vi "View.vi"(8 "error in (no error)":errorcluster) -> (0 "error out":errorcluster)   [LabVIEW 2019, in "STS_LTRV.lvlib"]
uses:
  STS_LTRV.lvlib
  Queue Driver/Queue Operation.ctl
  TypeDefs/Event Handler/Operation.ctl
  TypeDefs/UI Data.ctl
  TypeDefs/Publish Data.ctl
  TypeDefs/NumericLimit Data.ctl
  <vilib>/Utility/miscctls.llb/LVRowAndColumnTypeDef.ctl
  Queue Driver/Queue Driver.lvlib
panel:
  in  "Group Results by UUT":bool=TRUE
  in  "Max UUTs to Store":i32
  out "Diaplay Table":string[][](table)
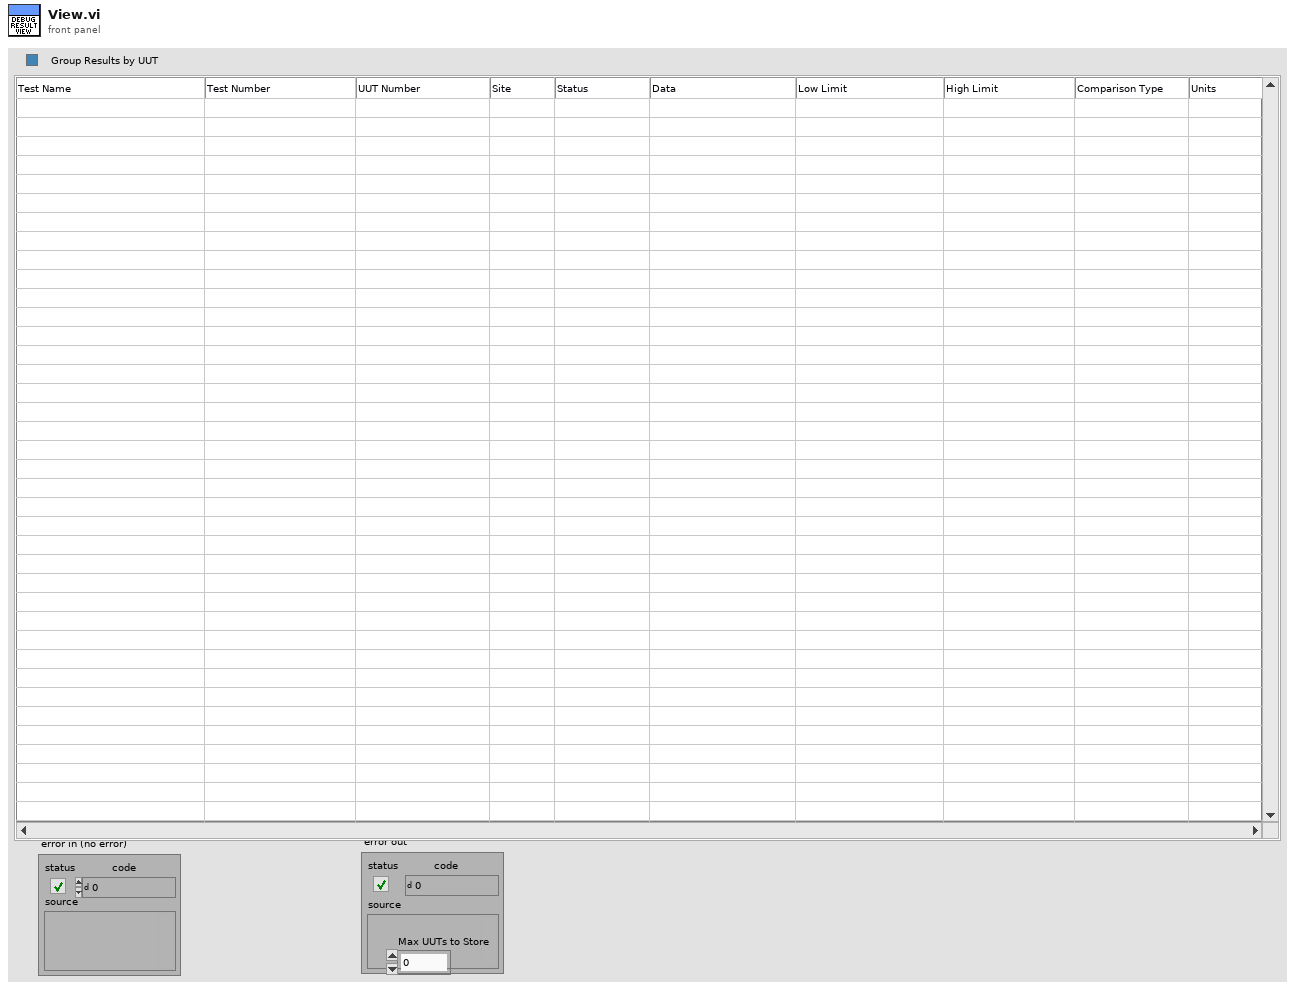
[diagram p1: front panel]
types:
  T1 = typedef "STS_LTRV.lvlib/UI Data.ctl" = cluster{"Order":u64, "Publish Data":T2}
  T2 = typedef "STS_LTRV.lvlib/Publish Data.ctl" = cluster{"TestName":string, "TestNumber":dbl, "Status":string, "UUT.SerialNumber":string, "Site":dbl, "NumericLimit":T3}
  T3 = typedef "STS_LTRV.lvlib/NumericLimit Data.ctl" = cluster{"Data":dbl, "LowLimit":dbl, "HighLimit":dbl, "ComparisonType":string, "Units":string}
  T4 = typedef "STS_LTRV.lvlib/Operation.ctl" = enum16{"Initilize", "Get Reference", "Publish", "Destroy"}
  T5 = cluster{"Data":variant, "Next Order Id":u64, "Max UUTs to Store":i32, "Group Results by UUT":bool}
  T6 = typedef "Queue Driver.lvlib/Queue Operation.ctl" = enum16{"Create", "Enqueue", "EnqueueN", "Dequeue", "Flush", "Destroy"}
  T7 = typedef "LVRowAndColumnTypeDef.ctl" = cluster{"Row":i32, "Column":i32}
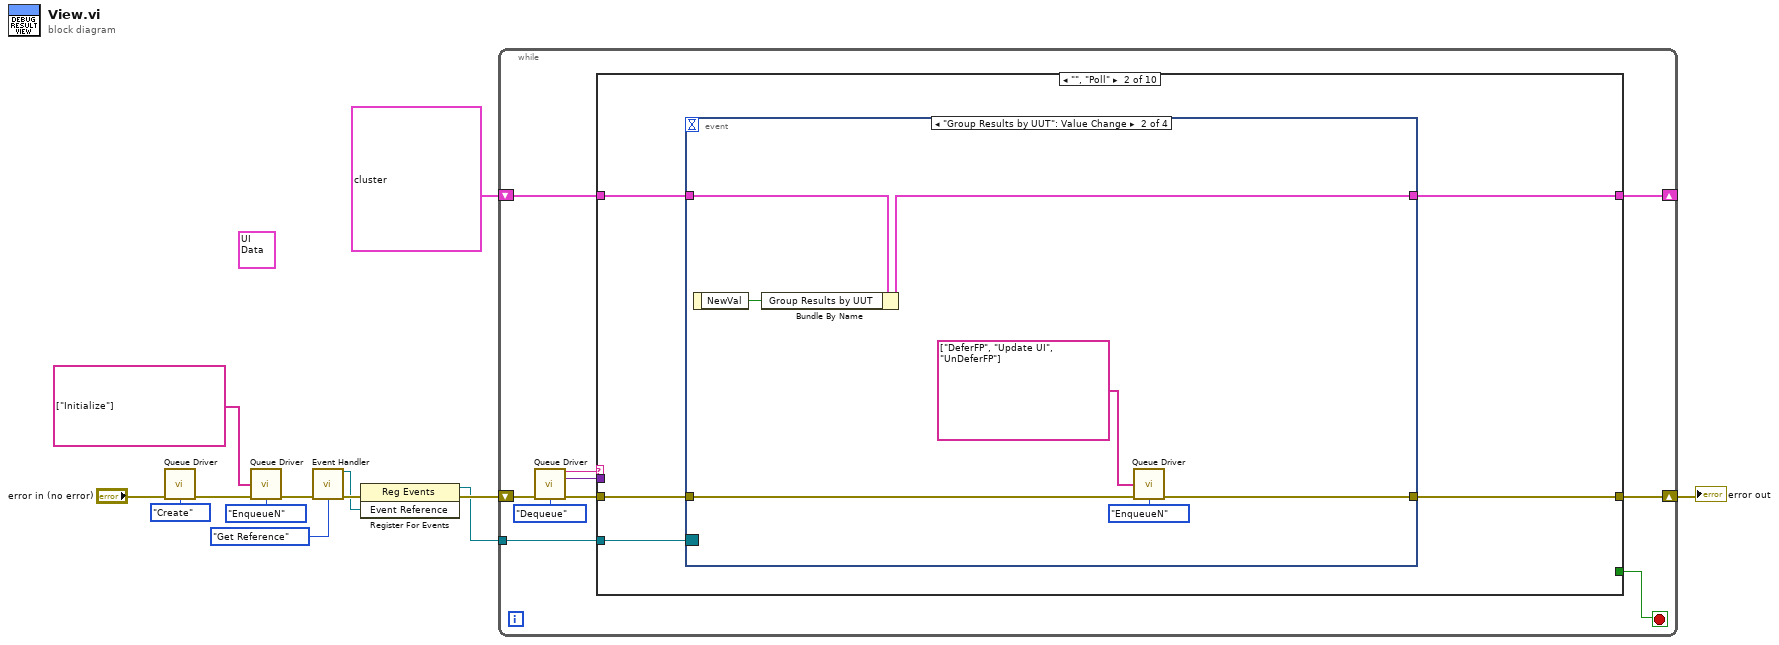
[diagram p0: block diagram]
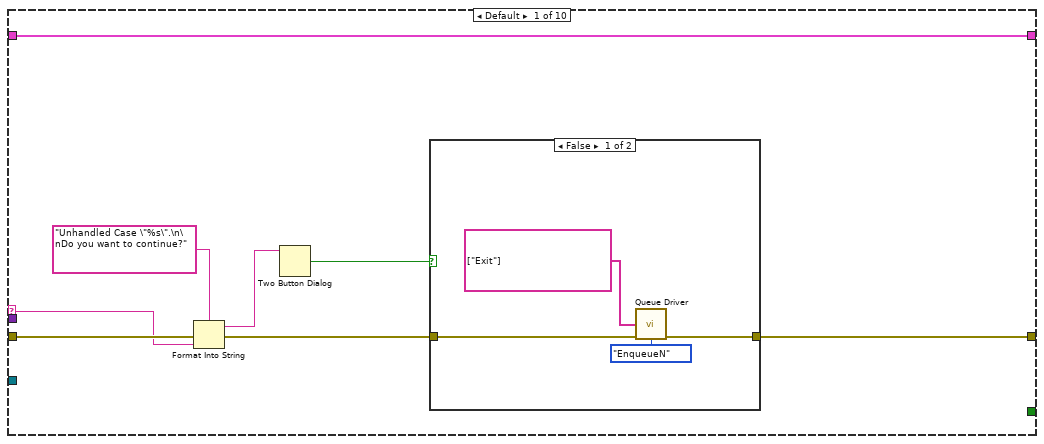
[diagram p2: hidden frame]
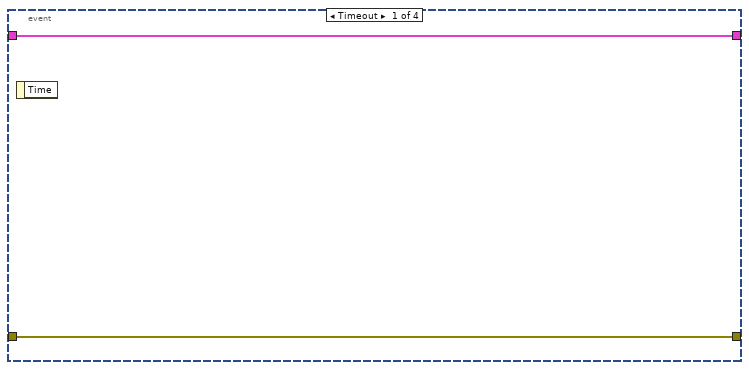
[diagram p4: hidden frame]
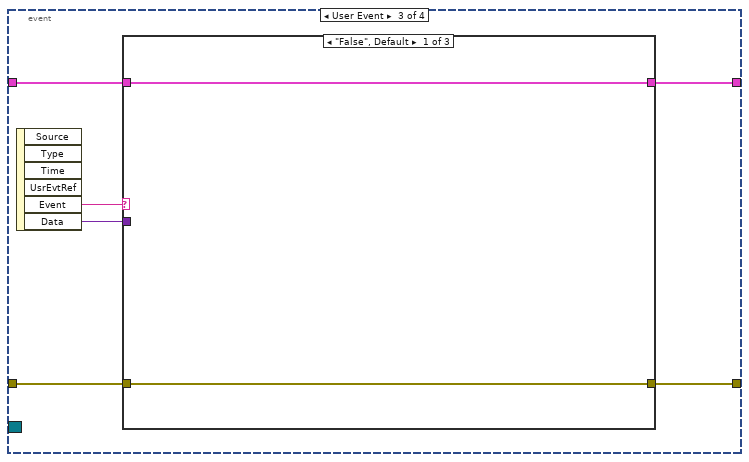
[diagram p5: hidden frame]
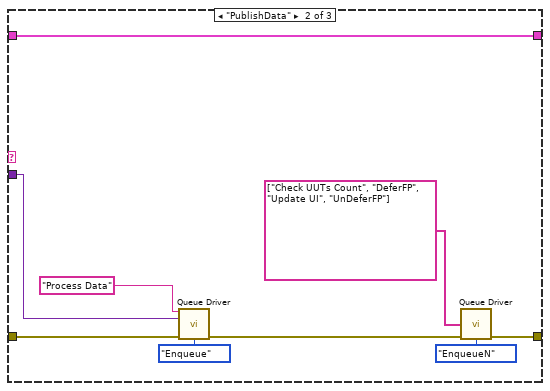
[diagram p6: hidden frame]
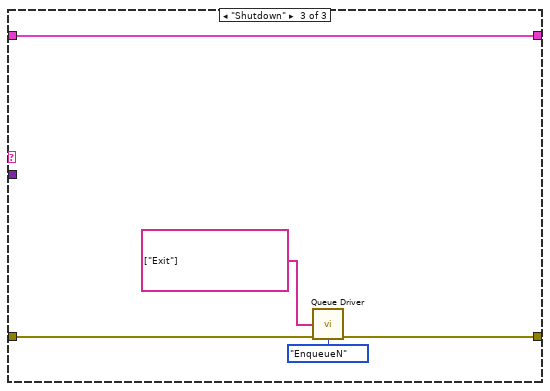
[diagram p7: hidden frame]
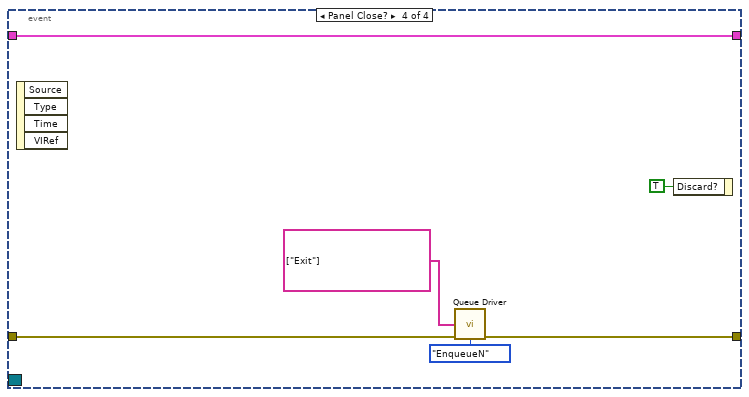
[diagram p8: hidden frame]
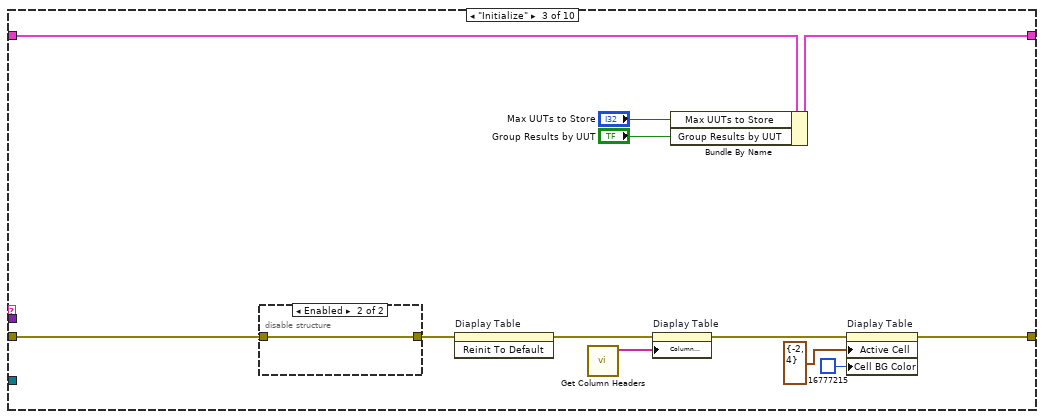
[diagram p9: hidden frame]
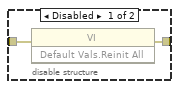
[diagram p10: hidden frame]
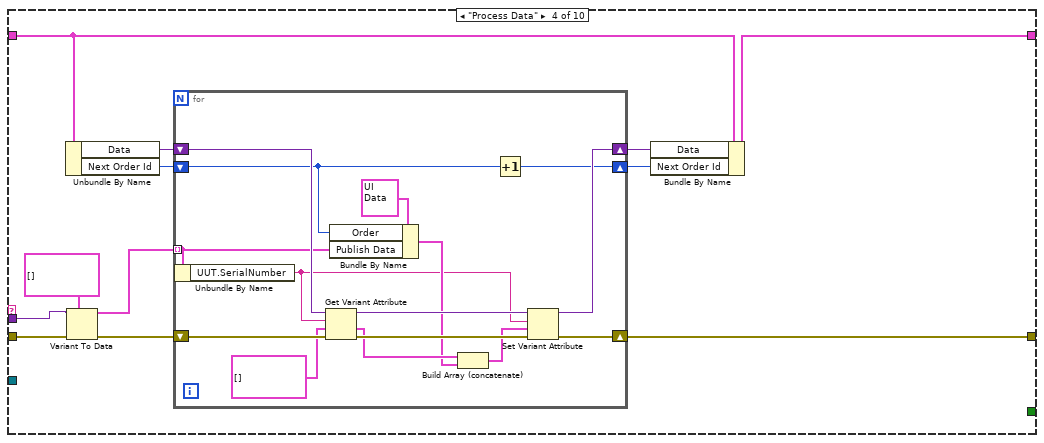
[diagram p11: hidden frame]
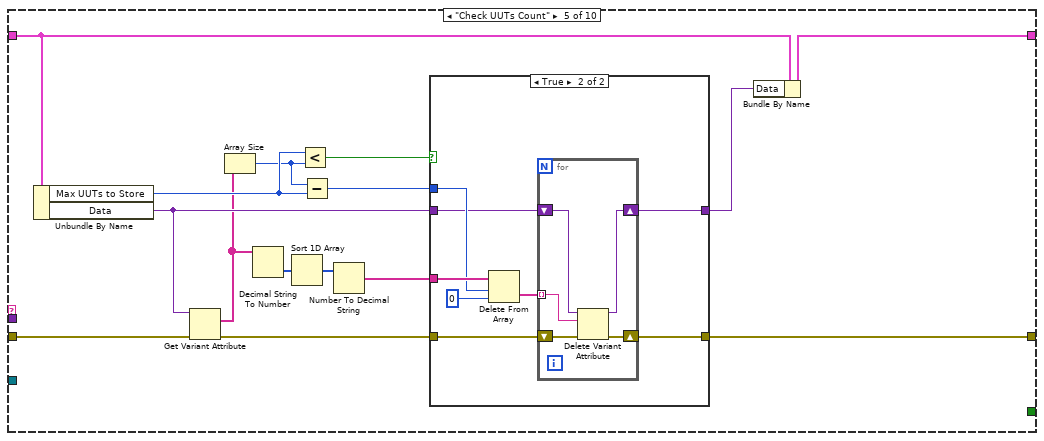
[diagram p12: hidden frame]
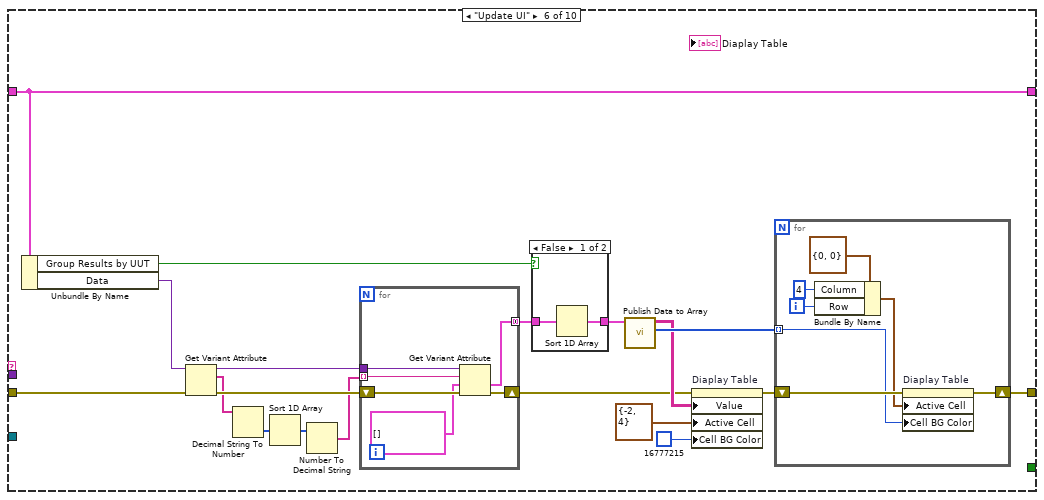
[diagram p14: hidden frame]
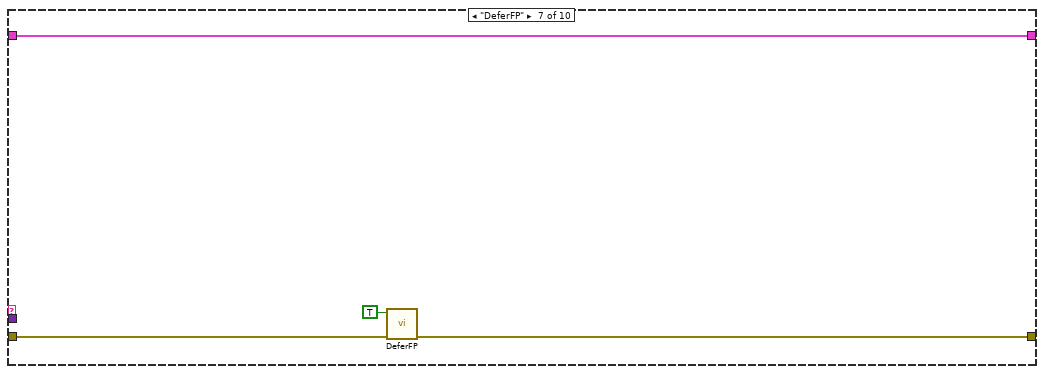
[diagram p16: hidden frame]
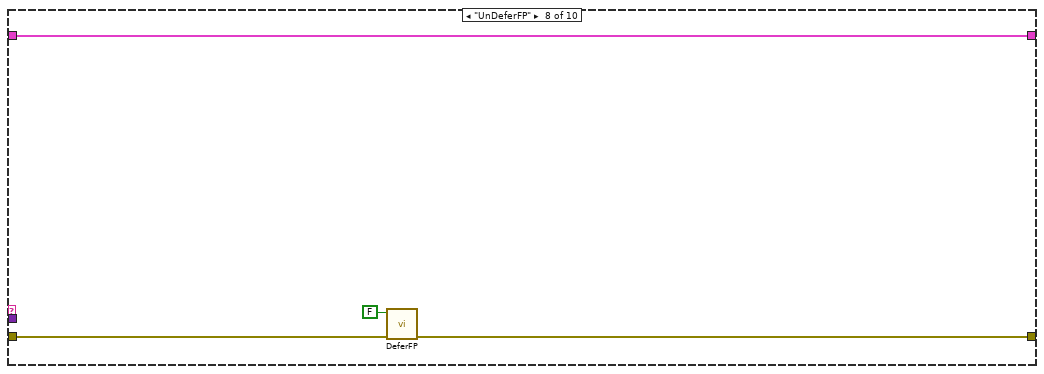
[diagram p17: hidden frame]
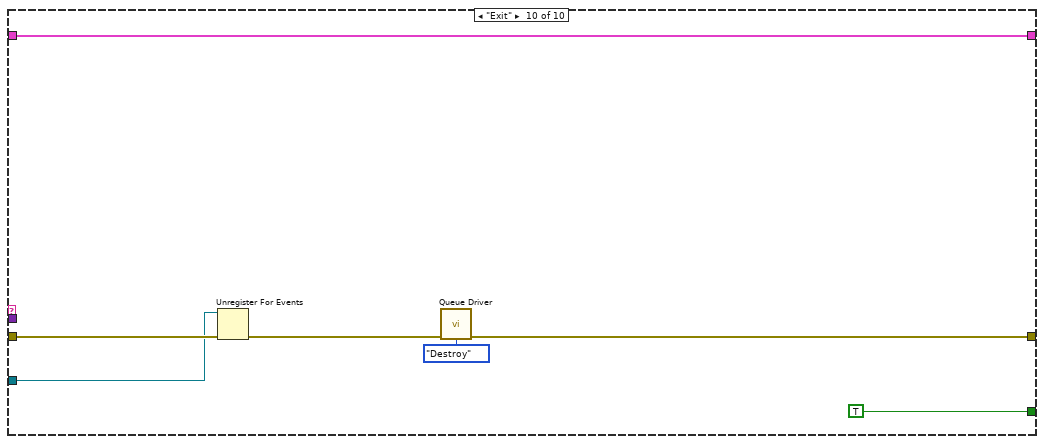
[diagram p19: hidden frame]
diagram:
  (unwired) T1 {"Order"=0, "Publish Data"={"TestName"="", "TestNumber"=0.0, "Status"="", "UUT.SerialNumber"="", "Site"=0.0, "NumericLimit"={"Data"=0.0, "LowLimit"=0.0, "HighLimit"=0.0, "ComparisonType"="", "Units"=""}}}
  n1 = call "Queue Driver.vi"("error in (no error)"="error in (no error)", "Queue Operation"=Queue_Operation."Create") -> ("error out"=w10:errorcluster)  [unwired: 11 in, 2 out]
  n2 = call "Queue Driver.vi"("EnqueueN States"=string[] ["Initialize"], "error in (no error)"=w10, "Queue Operation"=Queue_Operation."EnqueueN") -> ("error out"=w6:errorcluster)  [unwired: 10 in, 2 out]
  n3 = call "Event Handler.vi"("error in (no error)"=w6, "Operation"=Operation."Get Reference") -> ("Event Reference"=w2:refnum<user-event>, "error out"=w4:errorcluster)  [unwired: 12 in]
  n4 = register-events(error in=w4, w2) -> (reference out=w1:refnum<event-registration>, error out=w3:errorcluster)  [unwired: 1 in]
  n5 = while {
    shift-right: [w17] -> _
    shift-left: T5 {"Data"=variant, "Next Order Id"=0, "Max UUTs to Store"=0, "Group Results by UUT"=FALSE} -> [w19]
    shift-right: [w18] -> w7
    shift-left: w3 -> [w22]
    tunnel: w1 -> [w15]
    stop <- w16 stop-if-true
    n6 = call "Queue Driver.vi"("error in (no error)"=w22, "Queue Operation"=Queue_Operation."Dequeue") -> ("State Out"=w20:string, "Data Out"=w14:variant, "error out"=w21:errorcluster)  [unwired: 11 in]
    n7 = case shown="\"\", \"Poll\"" w20 {
      selector: w20 -> [w29 _ _ _ _ _ _ _ _ _]
      tunnel: w21 -> [w30 w41 w90 w105 w135 w168 w186 w190 w195 w197]
      tunnel: w19 -> [w31 w40 w86 w94 w127 w169 w189 w193 w194 w202]
      tunnel: [w25 w39 w80 w101 w130 w156 w187 w191 w195 w200] -> w18
      tunnel: [w31 w38 w87 w95 w128 w169 w189 w193 w194 w202] -> w17
      tunnel: [_ _ _ _ _ _ _ _ _ TRUE] -> w16
      tunnel: w15 -> [_ w37 _ _ _ _ _ _ _ w196]
      tunnel: w14 -> [_ _ _ w104 _ _ _ _ _ _]
      frame Default {
        n8 = Format Into String(format string="Unhandled Case \"%s\".\n\nDo you want to continue?", error in=w30, w29) -> (resulting string=w27:string, error out=w26:errorcluster)  [unwired: 1 in]
        n9 = Two Button Dialog(message=w27) -> (T button?=w24:bool)  [unwired: 2 in]
        n10 = case shown="False" w24 {
          tunnel: w26 -> [w34 w36]
          tunnel: [w33 w36] -> w25
          frame False {
            n11 = call "Queue Driver.vi"("EnqueueN States"=string[] ["Exit"], "error in (no error)"=w34, "Queue Operation"=Queue_Operation."EnqueueN") -> ("error out"=w33:errorcluster)  [unwired: 10 in, 2 out]
          }
          frame True {
          }
        }
      }
      frame "", "Poll" {
        n12 = event shown="[1] \"Group Results by UUT\": Value Change" {
          selector: w37 -> [_ _ _ _]
          dyn-events: _ -> [_ _ _ _]
          timeout: _ -> [_ _ _ _]
          tunnel: w41 -> [w43 w44 w55 w73]
          tunnel: w40 -> [w42 w49 w52 w78]
          tunnel: [w43 w45 w56 w74] -> w39
          tunnel: [w42 w50 w51 w78] -> w38
          event Timeout {
            n13 = event-data() -> ()  [unwired: 1 in, 1 out]
          }
          event "Group Results by UUT": Value Change {
            n14 = event-data() -> ("NewVal"=w48:bool)  [unwired: 1 in]
            n15 = Bundle By Name(cluster=w49, "Group Results by UUT"=w48) -> (w50:T5)
            n16 = call "Queue Driver.vi"("EnqueueN States"=string[] ["DeferFP", "Update UI", "UnDeferFP"], "error in (no error)"=w44, "Queue Operation"=Queue_Operation."EnqueueN") -> ("error out"=w45:errorcluster)  [unwired: 10 in, 2 out]
          }
          event User Event {
            n17 = event-data() -> ("Event"=w54:string, "Data"=w53:variant)  [unwired: 1 in, 4 out]
            n18 = case shown="\"False\", Default" w54 {
              tunnel: [w58 w65 w70] -> w56
              tunnel: w55 -> [w58 w62 w69]
              tunnel: w53 -> [_ w60 _]
              tunnel: w52 -> [w57 w64 w68]
              tunnel: [w57 w64 w68] -> w51
              frame "False", Default {
              }
              frame "PublishData" {
                n19 = call "Queue Driver.vi"("State In"="Process Data", "Data In"=w60, "error in (no error)"=w62, "Queue Operation"=Queue_Operation."Enqueue") -> ("error out"=w61:errorcluster)  [unwired: 9 in, 2 out]
                n20 = call "Queue Driver.vi"("EnqueueN States"=string[] ["Check UUTs Count", "DeferFP", "Update UI", "UnDeferFP"], "error in (no error)"=w61, "Queue Operation"=Queue_Operation."EnqueueN") -> ("error out"=w65:errorcluster)  [unwired: 10 in, 2 out]
              }
              frame "Shutdown" {
                n21 = call "Queue Driver.vi"("EnqueueN States"=string[] ["Exit"], "error in (no error)"=w69, "Queue Operation"=Queue_Operation."EnqueueN") -> ("error out"=w70:errorcluster)  [unwired: 10 in, 2 out]
              }
            }
          }
          event Panel Close? {
            n22 = event-data() -> ()  [unwired: 1 in, 4 out]
            n23 = call "Queue Driver.vi"("EnqueueN States"=string[] ["Exit"], "error in (no error)"=w73, "Queue Operation"=Queue_Operation."EnqueueN") -> ("error out"=w74:errorcluster)  [unwired: 10 in, 2 out]
            n24 = event-data("Discard?"=TRUE) -> ()  [unwired: 1 in, 1 out]
          }
        }
      }
      frame "Initialize" {
        n25 = disable-structure shown="Enabled" {
          disable-tunnel: w90 -> [w92 w93]
          disable-tunnel: [w91 w93] -> w89
          frame Disabled {
            n26 = invoke class="VI" method="Default Vals.Reinit All"(error in=w92) -> (error out=w91:errorcluster)  [unwired: 2 in, 2 out]
          }
          frame Enabled {
          }
        }
        n27 = invoke on="Diaplay Table" class="Tbl (strict)" method="Reinit To Default"(error in=w89) -> (error out=w84:errorcluster)  [unwired: 2 in, 2 out]
        n28 = call "Get Column Headers.vi"() -> ("Headers"=w85:string[])  [unwired: 11 in]
        n29 = property on="Diaplay Table" class="Tbl (strict)"(error in=w84, "Column Headers[]"=w85) -> (error out=w81:errorcluster)  [unwired: 1 in, 1 out]
        n30 = Bundle By Name(cluster=w86, "Max UUTs to Store"="Max UUTs to Store", "Group Results by UUT"="Group Results by UUT") -> (w87:T5)
        n31 = property on="Diaplay Table" class="Tbl (strict)"(error in=w81, "Active Cell"=T7 {"Row"=-2, "Column"=4} ("Active Cell:Active Cell"), "Cell BG Color"=u32 16777215) -> (error out=w80:errorcluster)  [unwired: 1 in, 1 out]
      }
      frame "Process Data" {
        n32 = Unbundle By Name(w94) -> ("Data"=w100:variant, "Next Order Id"=w98:u64)
        n33 = Variant To Data(error in=w105, type=T2[] [] ("Unprocessed Data"), Variant=w104) -> (data=w99:T2[], error out=w102:errorcluster)
        n34 = for {
          shift-right: [w116] -> w101
          shift-left: w102 -> [w120]
          tunnel: w99 -> [w112] mode=indexing
          shift-right: [w108] -> w97
          shift-left: w100 -> [w119]
          shift-right: [w107] -> w96
          shift-left: w98 -> [w113]
          n35 = Unbundle By Name(w112) -> ("UUT.SerialNumber"=w106:string)
          n36 = Get Variant Attribute(Variant=w119, name=w106, default value (empty Variant)=T1[] [], error in=w120) -> (duplicate Variant=w115:variant, value=w111:T1[], error out=w117:errorcluster)  [unwired: 1 out]
          n37 = Bundle By Name(cluster=T1 {"Order"=0, "Publish Data"={"TestName"="", "TestNumber"=0.0, "Status"="", "UUT.SerialNumber"="", "Site"=0.0, "NumericLimit"={"Data"=0.0, "LowLimit"=0.0, "HighLimit"=0.0, "ComparisonType"="", "Units"=""}}} ("Cluster"), "Order"=w113, "Publish Data"=w112) -> (w110:T1)
          n38 = Build Array (concatenate)(w111, w110) -> (w109:T1[])
          n39 = Increment(x=w113) -> (x+1=w107:u64)
          n40 = Set Variant Attribute(Variant=w115, name=w106, value=w109, error in=w117) -> (Variant out=w108:variant, error out=w116:errorcluster)  [unwired: 1 out]
        }
        n41 = Bundle By Name(cluster=w94, "Data"=w97, "Next Order Id"=w96) -> (w95:T5)
      }
      frame "Check UUTs Count" {
        n42 = Unbundle By Name(w127) -> ("Max UUTs to Store"=w134:i32, "Data"=w129:variant)
        n43 = Get Variant Attribute(Variant=w129, error in=w135) -> (names=w124:string[], error out=w131:errorcluster)  [unwired: 2 in, 2 out]
        n44 = Array Size(array=w124) -> (size(s)=w133:i32)
        n45 = Decimal String To Number(string=w124) -> (number=w123:i32[])  [unwired: 2 in, 1 out]
        n46 = Sort 1D Array(array=w123) -> (sorted array=w122:i32[])
        n47 = Less?(x=w134, y=w133) -> (x < y?=w125:bool)
        n48 = Subtract(x=w133, y=w134) -> (x-y=w132:i32)
        n49 = Number To Decimal String(number=w122) -> (decimal integer string=w121:string[])  [unwired: 1 in]
        n50 = case shown="True" w125 {
          tunnel: w121 -> [_ w145]
          tunnel: w132 -> [_ w144]
          tunnel: w131 -> [w137 w142]
          tunnel: [w137 w141] -> w130
          tunnel: w129 -> [w136 w140]
          tunnel: [w136 w138] -> w126
          frame False {
          }
          frame True {
            n51 = Delete From Array(array=w145, length=w144, index=0) -> (deleted portion=w139:string[])  [unwired: 1 out]
            n52 = for {
              shift-right: [w149] -> w141
              shift-left: w142 -> [w150]
              shift-right: [w146] -> w138
              shift-left: w140 -> [w148]
              tunnel: w139 -> [w147] mode=indexing
              n53 = Delete Variant Attribute(4:w150, 6:w147, 7:w148) -> (0:w149:errorcluster, 3:w146:variant)  [unwired: 1 out]
            }
          }
        }
        n54 = Bundle By Name(cluster=w127, "Data"=w126) -> (w128:T5)
      }
      frame "Update UI" {
        n55 = Unbundle By Name(w169) -> ("Group Results by UUT"=w155:bool, "Data"=w167:variant)
        n56 = Get Variant Attribute(Variant=w167, error in=w168) -> (duplicate Variant=w165:variant, names=w154:string[], error out=w166:errorcluster)  [unwired: 2 in, 1 out]
        n57 = Decimal String To Number(string=w154) -> (number=w153:i32[])  [unwired: 2 in, 1 out]
        n58 = Sort 1D Array(array=w153) -> (sorted array=w152:i32[])
        n59 = Number To Decimal String(number=w152) -> (decimal integer string=w151:string[])  [unwired: 1 in]
        n60 = for {
          shift-right: [w184] -> w157
          shift-left: w166 -> [w185]
          tunnel: w165 -> [w183]
          tunnel: w151 -> [w182] mode=indexing
          tunnel: [w180] -> w164 mode=concatenating
          n61 = Get Variant Attribute(Variant=w183, name=w182, default value (empty Variant)=T1[] [], error in=w185) -> (value=w180:T1[], error out=w184:errorcluster)  [unwired: 2 out]
        }
        n62 = case shown="False" w155 {
          tunnel: w164 -> [w171 w172]
          tunnel: [w170 w172] -> w163
          frame False {
            n63 = Sort 1D Array(array=w171) -> (sorted array=w170:T1[])
          }
          frame True {
          }
        }
        n64 = call "Publish Data to Array.vi"("Publish Data"=w163) -> ("Status Color"=w162:u32[], "Data[]"=w158:string[][])  [unwired: 9 in]
        n65 = property on="Diaplay Table" class="Tbl (strict)"(error in=w157, "Value"=w158, "Active Cell"=T7 {"Row"=-2, "Column"=4} ("Active Cell:Active Cell"), "Cell BG Color"=u32 16777215) -> (error out=w161:errorcluster)  [unwired: 1 in, 1 out]
        n66 = for {
          shift-right: [w178] -> w156
          shift-left: w161 -> [w179]
          tunnel: w162 -> [w174] mode=indexing
          i -> [w173]
          n67 = Bundle By Name(cluster=T7 {"Row"=0, "Column"=0} ("Active Cell:Active Cell"), "Column"=4, "Row"=w173) -> (w176:T7)
          n68 = property on="Diaplay Table" class="Tbl (strict)"(error in=w179, "Active Cell"=w176, "Cell BG Color"=w174) -> (error out=w178:errorcluster)  [unwired: 1 in, 1 out]
        }
      }
      frame "DeferFP" {
        n69 = call "DeferFP.vi"("error in"=w186, "Defer Front Panel?"=TRUE) -> ("error out"=w187:errorcluster)  [unwired: 9 in]
      }
      frame "UnDeferFP" {
        n70 = call "DeferFP.vi"("error in"=w190, "Defer Front Panel?"=FALSE) -> ("error out"=w191:errorcluster)  [unwired: 9 in]
      }
      frame "Error" {
      }
      frame "Exit" {
        n71 = Unregister For Events(event registration refnum=w196, error in=w197) -> (error out=w198:errorcluster)
        n72 = call "Queue Driver.vi"("error in (no error)"=w198, "Queue Operation"=Queue_Operation."Destroy") -> ("error out"=w200:errorcluster)  [unwired: 11 in, 2 out]
      }
    }
  }
  "error out" <- w7
